vi "Pumps_Valves_Dependencies.vi"(8 "Set state:":bool, 10 "Device":T1=enum."V7") -> (0 "State":bool)   [LabVIEW 2011]
uses:
  Valve_Pump.ctl
  Pumps_Valves_Dependencies_Global.vi
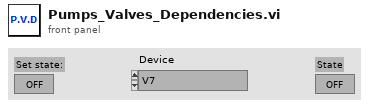
[diagram p1: front panel]
types:
  T1 = typedef "Valve_Pump.ctl" = enum16{"Main Rack Power", "Pump Power", "Valve Power", "V4", "V5", "V6", "V7", "V8", "V9", "V10", "V11", "V12", "V13", "V14", "V15", "V18", "V19", "V20", "V21", "V22", "V23", "V24", "V25", "V26", "V27", "V28", "V29", "V30", "V31", "V32", "V33", "V34", "Pump A", "Pump B", "Pump C", "Pump D"}
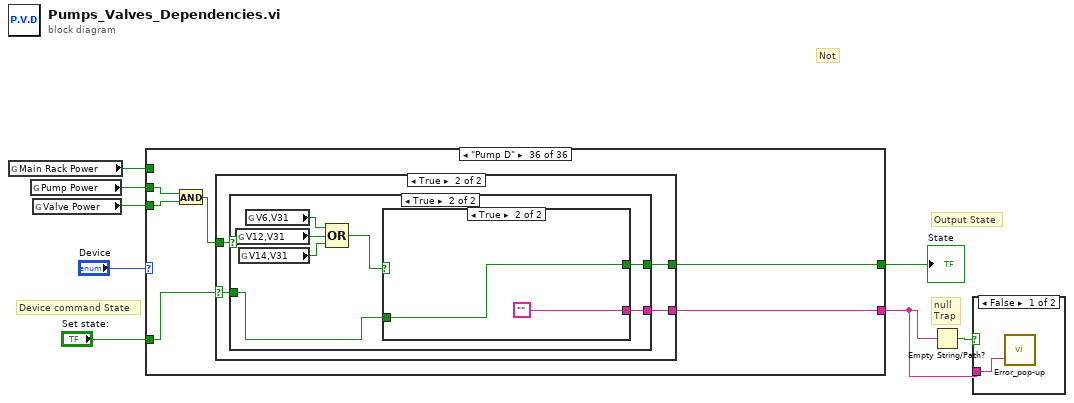
[diagram p0: block diagram]
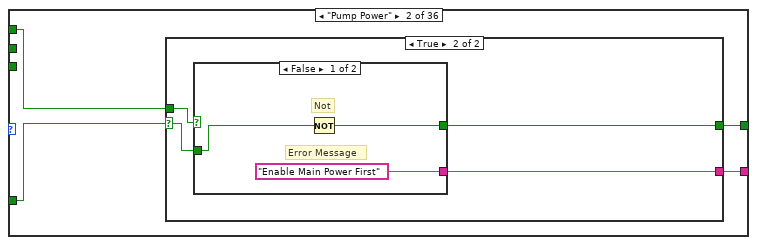
[diagram p4: hidden frame]
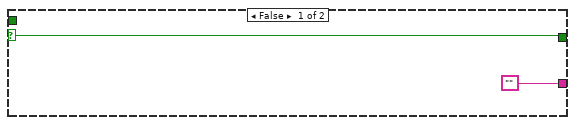
[diagram p5: hidden frame]
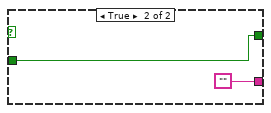
[diagram p6: hidden frame]
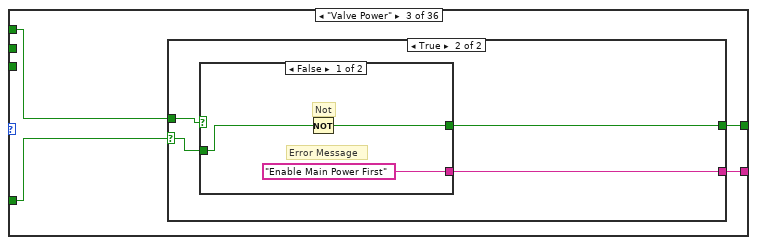
[diagram p7: hidden frame]
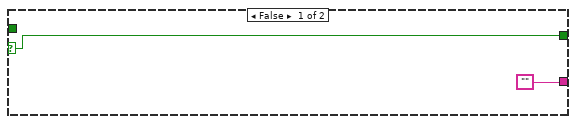
[diagram p8: hidden frame]
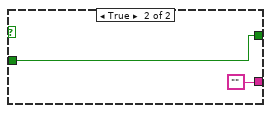
[diagram p9: hidden frame]
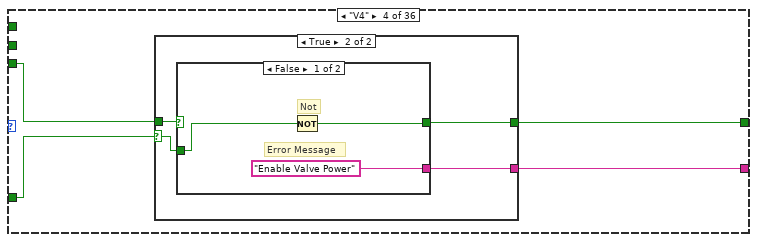
[diagram p10: hidden frame]
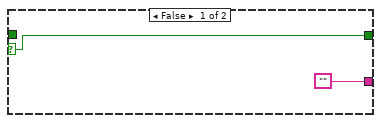
[diagram p11: hidden frame]
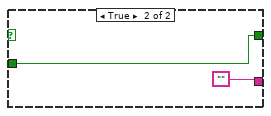
[diagram p12: hidden frame]
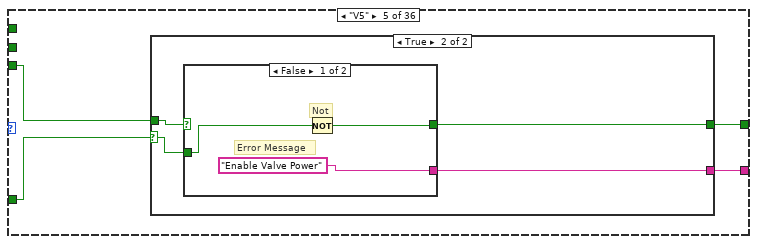
[diagram p13: hidden frame]
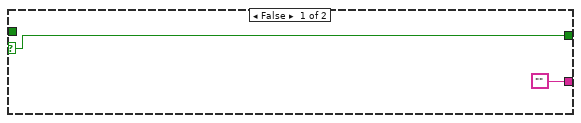
[diagram p14: hidden frame]
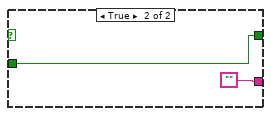
[diagram p15: hidden frame]
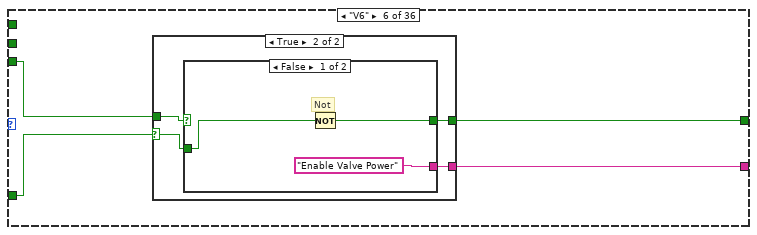
[diagram p16: hidden frame]
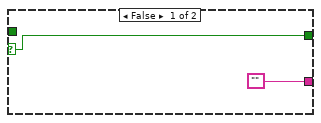
[diagram p17: hidden frame]
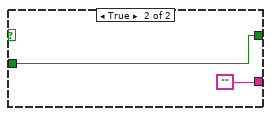
[diagram p18: hidden frame]
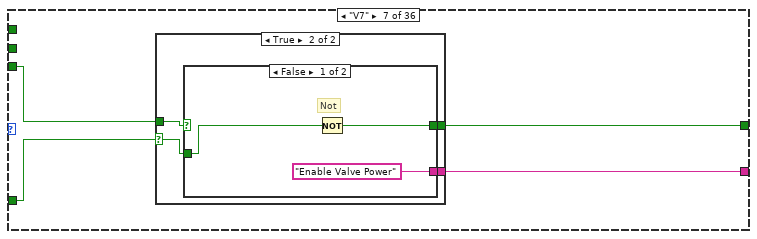
[diagram p19: hidden frame]
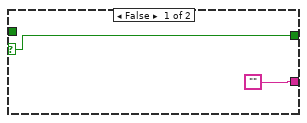
[diagram p20: hidden frame]
diagram:
  # "null\nTrap"
  # "Not"
  # "Device command State"
  # "Output State"
  n1 = global read "Pumps_Valves_Dependencies_Global.vi" "Main Rack Power"() -> (w3:bool)
  n2 = global read "Pumps_Valves_Dependencies_Global.vi" "Pump Power"() -> (w2:bool)
  n3 = global read "Pumps_Valves_Dependencies_Global.vi" "Valve Power"() -> (w1:bool)
  n4 = case shown="\"Pump D\"" "Device" {
    tunnel: "Set state:" -> [w9 w10 w25 w40 w55 w70 w85 w100 w115 w130 w145 w160 w175 w190 w205 w220 w235 w250 w265 w280 w295 w310 w325 w340 w355 w370 w385 w400 w415 w430 w445 w460 w475 w503 w530 w556]
    tunnel: [w9 w13 w27 w43 w58 w73 w88 w103 w118 w133 w148 w163 w178 w193 w208 w223 w238 w253 w268 w283 w298 w313 w328 w343 w358 w373 w388 w403 w418 w433 w448 w463 w477 w508 w533 w558] -> w6
    tunnel: [_ w12 w28 w42 w57 w72 w87 w102 w117 w132 w147 w162 w177 w192 w207 w222 w237 w252 w267 w282 w297 w312 w327 w342 w357 w372 w387 w402 w417 w432 w447 w462 w480 w507 w532 w559] -> w4
    tunnel: w3 -> [_ w11 w26 _ _ _ _ _ _ _ _ _ _ _ _ _ _ _ _ _ _ _ _ _ _ _ _ _ _ _ _ _ _ _ _ _]
    tunnel: w2 -> [_ _ _ _ _ _ _ _ _ _ _ _ _ _ _ _ _ _ _ _ _ _ _ _ _ _ _ _ _ _ _ _ w478 w505 w535 w561]
    tunnel: w1 -> [_ _ _ w41 w56 w71 w86 w101 w116 w131 w146 w161 w176 w191 w206 w221 w236 w251 w266 w281 w296 w311 w326 w341 w356 w371 w386 w401 w416 w431 w446 w461 w479 w506 w534 w560]
    frame "Main Rack Power" {
    }
    frame "Pump Power" {
      n5 = case shown="True" w10 {
        selector: w10 -> [w15 w16]
        tunnel: [w15 w19] -> w13
        tunnel: ["" w18] -> w12
        tunnel: w11 -> [_ w17]
        frame False {
        }
        frame True {
          n6 = case shown="False" w17 {
            tunnel: [w20 w24] -> w19
            tunnel: w16 -> [w21 w24]
            tunnel: ["Enable Main Power First" ""] -> w18
            frame False {
              # "Error Message"
              # "Not"
              n7 = Not(x=w21) -> (.not. x?=w20:bool)
            }
            frame True {
            }
          }
        }
      }
    }
    frame "Valve Power" {
      n8 = case shown="True" w25 {
        selector: w25 -> [w30 w31]
        tunnel: ["" w34] -> w28
        tunnel: [w30 w33] -> w27
        tunnel: w26 -> [_ w32]
        frame False {
        }
        frame True {
          n9 = case shown="False" w32 {
            tunnel: [w35 w39] -> w33
            tunnel: w31 -> [w36 w39]
            tunnel: ["Enable Main Power First" ""] -> w34
            frame False {
              # "Error Message"
              # "Not"
              n10 = Not(x=w36) -> (.not. x?=w35:bool)
            }
            frame True {
            }
          }
        }
      }
    }
    frame "V4" {
      n11 = case shown="True" w40 {
        selector: w40 -> [w45 w46]
        tunnel: [w45 w49] -> w43
        tunnel: ["" w48] -> w42
        tunnel: w41 -> [_ w47]
        frame False {
        }
        frame True {
          n12 = case shown="False" w47 {
            tunnel: [w50 w54] -> w49
            tunnel: w46 -> [w51 w54]
            tunnel: ["Enable Valve Power" ""] -> w48
            frame False {
              # "Not"
              # "Error Message"
              n13 = Not(x=w51) -> (.not. x?=w50:bool)
            }
            frame True {
            }
          }
        }
      }
    }
    frame "V5" {
      n14 = case shown="True" w55 {
        selector: w55 -> [w60 w61]
        tunnel: [w60 w64] -> w58
        tunnel: ["" w63] -> w57
        tunnel: w56 -> [_ w62]
        frame False {
        }
        frame True {
          n15 = case shown="False" w62 {
            tunnel: [w66 w69] -> w64
            tunnel: w61 -> [w65 w69]
            tunnel: ["Enable Valve Power" ""] -> w63
            frame False {
              # "Error Message"
              # "Not"
              n16 = Not(x=w65) -> (.not. x?=w66:bool)
            }
            frame True {
            }
          }
        }
      }
    }
    frame "V6" {
      n17 = case shown="True" w70 {
        selector: w70 -> [w75 w76]
        tunnel: [w75 w79] -> w73
        tunnel: ["" w78] -> w72
        tunnel: w71 -> [_ w77]
        frame False {
        }
        frame True {
          n18 = case shown="False" w77 {
            tunnel: [w81 w84] -> w79
            tunnel: w76 -> [w80 w84]
            tunnel: ["Enable Valve Power" ""] -> w78
            frame False {
              # "Not"
              n19 = Not(x=w80) -> (.not. x?=w81:bool)
            }
            frame True {
            }
          }
        }
      }
    }
    frame "V7" {
      n20 = case shown="True" w85 {
        selector: w85 -> [w90 w91]
        tunnel: [w90 w94] -> w88
        tunnel: ["" w93] -> w87
        tunnel: w86 -> [_ w92]
        frame False {
        }
        frame True {
          n21 = case shown="False" w92 {
            tunnel: [w96 w99] -> w94
            tunnel: w91 -> [w95 w99]
            tunnel: ["Enable Valve Power" ""] -> w93
            frame False {
              # "Not"
              n22 = Not(x=w95) -> (.not. x?=w96:bool)
            }
            frame True {
            }
          }
        }
      }
    }
    frame "V8" {
      n23 = case shown="True" w100 {
        selector: w100 -> [w104 w106]
        tunnel: [w104 w109] -> w103
        tunnel: ["" w108] -> w102
        tunnel: w101 -> [_ w107]
        frame False {
        }
        frame True {
          n24 = case shown="False" w107 {
            tunnel: [w110 w114] -> w109
            tunnel: w106 -> [w111 w114]
            tunnel: ["Enable Valve Power" ""] -> w108
            frame False {
              # "Not"
              n25 = Not(x=w111) -> (.not. x?=w110:bool)
            }
            frame True {
            }
          }
        }
      }
    }
    frame "V9" {
      n26 = case shown="True" w115 {
        selector: w115 -> [w120 w121]
        tunnel: [w120 w124] -> w118
        tunnel: ["" w123] -> w117
        tunnel: w116 -> [_ w122]
        frame False {
        }
        frame True {
          n27 = case shown="False" w122 {
            tunnel: [w126 w129] -> w124
            tunnel: w121 -> [w125 w129]
            tunnel: ["Enable Valve Power" ""] -> w123
            frame False {
              # "Not"
              n28 = Not(x=w125) -> (.not. x?=w126:bool)
            }
            frame True {
            }
          }
        }
      }
    }
    frame "V10" {
      n29 = case shown="True" w130 {
        selector: w130 -> [w135 w136]
        tunnel: [w135 w139] -> w133
        tunnel: ["" w138] -> w132
        tunnel: w131 -> [_ w137]
        frame False {
        }
        frame True {
          n30 = case shown="False" w137 {
            tunnel: [w140 w144] -> w139
            tunnel: w136 -> [w141 w144]
            tunnel: ["Enable Valve Power" ""] -> w138
            frame False {
              # "Not"
              n31 = Not(x=w141) -> (.not. x?=w140:bool)
            }
            frame True {
            }
          }
        }
      }
    }
    frame "V11" {
      n32 = case shown="True" w145 {
        selector: w145 -> [w150 w151]
        tunnel: [w150 w154] -> w148
        tunnel: ["" w153] -> w147
        tunnel: w146 -> [_ w152]
        frame False {
        }
        frame True {
          n33 = case shown="False" w152 {
            tunnel: [w155 w159] -> w154
            tunnel: w151 -> [w156 w159]
            tunnel: ["Enable Valve Power" ""] -> w153
            frame False {
              # "Not"
              n34 = Not(x=w156) -> (.not. x?=w155:bool)
            }
            frame True {
            }
          }
        }
      }
    }
    frame "V12" {
      n35 = case shown="True" w160 {
        selector: w160 -> [w164 w166]
        tunnel: [w164 w169] -> w163
        tunnel: ["" w168] -> w162
        tunnel: w161 -> [_ w167]
        frame False {
        }
        frame True {
          n36 = case shown="False" w167 {
            tunnel: [w171 w174] -> w169
            tunnel: w166 -> [w170 w174]
            tunnel: ["Enable Valve Power" ""] -> w168
            frame False {
              # "Not"
              n37 = Not(x=w170) -> (.not. x?=w171:bool)
            }
            frame True {
            }
          }
        }
      }
    }
    frame "V13" {
      n38 = case shown="True" w175 {
        selector: w175 -> [w180 w181]
        tunnel: [w180 w184] -> w178
        tunnel: ["" w183] -> w177
        tunnel: w176 -> [_ w182]
        frame False {
        }
        frame True {
          n39 = case shown="False" w182 {
            tunnel: [w186 w189] -> w184
            tunnel: w181 -> [w185 w189]
            tunnel: ["Enable Valve Power" ""] -> w183
            frame False {
              # "Not"
              n40 = Not(x=w185) -> (.not. x?=w186:bool)
            }
            frame True {
            }
          }
        }
      }
    }
    frame "V14" {
      n41 = case shown="True" w190 {
        selector: w190 -> [w194 w196]
        tunnel: [w194 w199] -> w193
        tunnel: ["" w198] -> w192
        tunnel: w191 -> [_ w197]
        frame False {
        }
        frame True {
          n42 = case shown="False" w197 {
            tunnel: [w200 w204] -> w199
            tunnel: w196 -> [w201 w204]
            tunnel: ["Enable Valve Power" ""] -> w198
            frame False {
              # "Not"
              n43 = Not(x=w201) -> (.not. x?=w200:bool)
            }
            frame True {
            }
          }
        }
      }
    }
    frame "V15" {
      n44 = case shown="True" w205 {
        selector: w205 -> [w210 w211]
        tunnel: [w210 w214] -> w208
        tunnel: ["" w213] -> w207
        tunnel: w206 -> [_ w212]
        frame False {
        }
        frame True {
          n45 = case shown="False" w212 {
            tunnel: [w215 w219] -> w214
            tunnel: w211 -> [w216 w219]
            tunnel: ["Enable Valve Power" ""] -> w213
            frame False {
              # "Not"
              n46 = Not(x=w216) -> (.not. x?=w215:bool)
            }
            frame True {
            }
          }
        }
      }
    }
    frame "V18" {
      n47 = case shown="True" w220 {
        selector: w220 -> [w225 w226]
        tunnel: [w225 w229] -> w223
        tunnel: ["" w228] -> w222
        tunnel: w221 -> [_ w227]
        frame False {
        }
        frame True {
          n48 = case shown="False" w227 {
            tunnel: [w231 w234] -> w229
            tunnel: w226 -> [w230 w234]
            tunnel: ["Enable Valve Power" ""] -> w228
            frame False {
              # "Not"
              n49 = Not(x=w230) -> (.not. x?=w231:bool)
            }
            frame True {
            }
          }
        }
      }
    }
    frame "V19" {
      n50 = case shown="True" w235 {
        selector: w235 -> [w240 w241]
        tunnel: [w240 w244] -> w238
        tunnel: ["" w243] -> w237
        tunnel: w236 -> [_ w242]
        frame False {
        }
        frame True {
          n51 = case shown="False" w242 {
            tunnel: [w246 w249] -> w244
            tunnel: w241 -> [w245 w249]
            tunnel: ["Enable Valve Power" ""] -> w243
            frame False {
              # "Not"
              n52 = Not(x=w245) -> (.not. x?=w246:bool)
            }
            frame True {
            }
          }
        }
      }
    }
    frame "V20" {
      n53 = case shown="True" w250 {
        selector: w250 -> [w255 w256]
        tunnel: [w255 w259] -> w253
        tunnel: ["" w258] -> w252
        tunnel: w251 -> [_ w257]
        frame False {
        }
        frame True {
          n54 = case shown="False" w257 {
            tunnel: [w261 w264] -> w259
            tunnel: w256 -> [w260 w264]
            tunnel: ["Enable Valve Power" ""] -> w258
            frame False {
              # "Not"
              n55 = Not(x=w260) -> (.not. x?=w261:bool)
            }
            frame True {
            }
          }
        }
      }
    }
    frame "V21" {
      n56 = case shown="True" w265 {
        selector: w265 -> [w270 w271]
        tunnel: [w270 w274] -> w268
        tunnel: ["" w273] -> w267
        tunnel: w266 -> [_ w272]
        frame False {
        }
        frame True {
          n57 = case shown="False" w272 {
            tunnel: [w276 w279] -> w274
            tunnel: w271 -> [w275 w279]
            tunnel: ["Enable Valve Power" ""] -> w273
            frame False {
              # "Not"
              n58 = Not(x=w275) -> (.not. x?=w276:bool)
            }
            frame True {
            }
          }
        }
      }
    }
    frame "V22" {
      n59 = case shown="True" w280 {
        selector: w280 -> [w285 w286]
        tunnel: [w285 w289] -> w283
        tunnel: ["" w288] -> w282
        tunnel: w281 -> [_ w287]
        frame False {
        }
        frame True {
          n60 = case shown="False" w287 {
            tunnel: [w291 w294] -> w289
            tunnel: w286 -> [w290 w294]
            tunnel: ["Enable Valve Power" ""] -> w288
            frame False {
              # "Not"
              n61 = Not(x=w290) -> (.not. x?=w291:bool)
            }
            frame True {
            }
          }
        }
      }
    }
    frame "V23" {
      n62 = case shown="True" w295 {
        selector: w295 -> [w300 w301]
        tunnel: [w300 w304] -> w298
        tunnel: ["" w303] -> w297
        tunnel: w296 -> [_ w302]
        frame False {
        }
        frame True {
          n63 = case shown="False" w302 {
            tunnel: [w306 w309] -> w304
            tunnel: w301 -> [w305 w309]
            tunnel: ["Enable Valve Power" ""] -> w303
            frame False {
              # "Not"
              n64 = Not(x=w305) -> (.not. x?=w306:bool)
            }
            frame True {
            }
          }
        }
      }
    }
    frame "V24" {
      n65 = case shown="True" w310 {
        selector: w310 -> [w315 w316]
        tunnel: [w315 w319] -> w313
        tunnel: ["" w318] -> w312
        tunnel: w311 -> [_ w317]
        frame False {
        }
        frame True {
          n66 = case shown="False" w317 {
            tunnel: [w321 w324] -> w319
            tunnel: w316 -> [w320 w324]
            tunnel: ["Enable Valve Power" ""] -> w318
            frame False {
              # "Not"
              n67 = Not(x=w320) -> (.not. x?=w321:bool)
            }
            frame True {
            }
          }
        }
      }
    }
    frame "V25" {
      n68 = case shown="True" w325 {
        selector: w325 -> [w330 w331]
        tunnel: [w330 w334] -> w328
        tunnel: ["" w333] -> w327
        tunnel: w326 -> [_ w332]
        frame False {
        }
        frame True {
          n69 = case shown="False" w332 {
            tunnel: [w336 w339] -> w334
            tunnel: w331 -> [w335 w339]
            tunnel: ["Enable Valve Power" ""] -> w333
            frame False {
              # "Not"
              n70 = Not(x=w335) -> (.not. x?=w336:bool)
            }
            frame True {
            }
          }
        }
      }
    }
    frame "V26" {
      n71 = case shown="True" w340 {
        selector: w340 -> [w345 w346]
        tunnel: [w345 w349] -> w343
        tunnel: ["" w348] -> w342
        tunnel: w341 -> [_ w347]
        frame False {
        }
        frame True {
          n72 = case shown="False" w347 {
            tunnel: [w351 w354] -> w349
            tunnel: w346 -> [w350 w354]
            tunnel: ["Enable Valve Power" ""] -> w348
            frame False {
              # "Not"
              n73 = Not(x=w350) -> (.not. x?=w351:bool)
            }
            frame True {
            }
          }
        }
      }
    }
    frame "V27" {
      n74 = case shown="True" w355 {
        selector: w355 -> [w360 w361]
        tunnel: [w360 w364] -> w358
        tunnel: ["" w363] -> w357
        tunnel: w356 -> [_ w362]
        frame False {
        }
        frame True {
          n75 = case shown="False" w362 {
            tunnel: [w366 w369] -> w364
            tunnel: w361 -> [w365 w369]
            tunnel: ["Enable Valve Power" ""] -> w363
            frame False {
              # "Not"
              n76 = Not(x=w365) -> (.not. x?=w366:bool)
            }
            frame True {
            }
          }
        }
      }
    }
    frame "V28" {
      n77 = case shown="True" w370 {
        selector: w370 -> [w375 w376]
        tunnel: [w375 w379] -> w373
        tunnel: ["" w378] -> w372
        tunnel: w371 -> [_ w377]
        frame False {
        }
        frame True {
          n78 = case shown="False" w377 {
            tunnel: [w381 w384] -> w379
            tunnel: w376 -> [w380 w384]
            tunnel: ["Enable Valve Power" ""] -> w378
            frame False {
              # "Not"
              n79 = Not(x=w380) -> (.not. x?=w381:bool)
            }
            frame True {
            }
          }
        }
      }
    }
    frame "V29" {
      n80 = case shown="True" w385 {
        selector: w385 -> [w390 w391]
        tunnel: [w390 w394] -> w388
        tunnel: ["" w393] -> w387
        tunnel: w386 -> [_ w392]
        frame False {
        }
        frame True {
          n81 = case shown="False" w392 {
            tunnel: [w396 w399] -> w394
            tunnel: w391 -> [w395 w399]
            tunnel: ["Enable Valve Power" ""] -> w393
            frame False {
              # "Not"
              n82 = Not(x=w395) -> (.not. x?=w396:bool)
            }
            frame True {
            }
          }
        }
      }
    }
    frame "V30" {
      n83 = case shown="True" w400 {
        selector: w400 -> [w405 w406]
        tunnel: [w405 w409] -> w403
        tunnel: ["" w408] -> w402
        tunnel: w401 -> [_ w407]
        frame False {
        }
        frame True {
          n84 = case shown="False" w407 {
            tunnel: [w411 w414] -> w409
            tunnel: w406 -> [w410 w414]
            tunnel: ["Enable Valve Power" ""] -> w408
            frame False {
              # "Not"
              n85 = Not(x=w410) -> (.not. x?=w411:bool)
            }
            frame True {
            }
          }
        }
      }
    }
    frame "V31" {
      n86 = case shown="True" w415 {
        selector: w415 -> [w420 w421]
        tunnel: [w420 w424] -> w418
        tunnel: ["" w423] -> w417
        tunnel: w416 -> [_ w422]
        frame False {
        }
        frame True {
          n87 = case shown="False" w422 {
            tunnel: [w426 w429] -> w424
            tunnel: w421 -> [w425 w429]
            tunnel: ["Enable Valve Power" ""] -> w423
            frame False {
              # "Not"
              n88 = Not(x=w425) -> (.not. x?=w426:bool)
            }
            frame True {
            }
          }
        }
      }
    }
    frame "V32" {
      n89 = case shown="True" w430 {
        selector: w430 -> [w435 w436]
        tunnel: [w435 w439] -> w433
        tunnel: ["" w438] -> w432
        tunnel: w431 -> [_ w437]
        frame False {
        }
        frame True {
          n90 = case shown="False" w437 {
            tunnel: [w441 w444] -> w439
            tunnel: w436 -> [w440 w444]
            tunnel: ["Enable Valve Power" ""] -> w438
            frame False {
              # "Not"
              n91 = Not(x=w440) -> (.not. x?=w441:bool)
            }
            frame True {
            }
          }
        }
      }
    }
    frame "V33" {
      n92 = case shown="True" w445 {
        selector: w445 -> [w450 w451]
        tunnel: [w450 w454] -> w448
        tunnel: ["" w453] -> w447
        tunnel: w446 -> [_ w452]
        frame False {
        }
        frame True {
          n93 = case shown="False" w452 {
            tunnel: [w456 w459] -> w454
            tunnel: w451 -> [w455 w459]
            tunnel: ["Enable Valve Power" ""] -> w453
            frame False {
              # "Not"
              n94 = Not(x=w455) -> (.not. x?=w456:bool)
            }
            frame True {
            }
          }
        }
      }
    }
    frame "V34" {
      n95 = case shown="True" w460 {
        selector: w460 -> [w465 w466]
        tunnel: [w465 w469] -> w463
        tunnel: ["" w468] -> w462
        tunnel: w461 -> [_ w467]
        frame False {
        }
        frame True {
          n96 = case shown="False" w467 {
            tunnel: [w471 w474] -> w469
            tunnel: w466 -> [w470 w474]
            tunnel: ["Enable Valve Power" ""] -> w468
            frame False {
              # "Not"
              n97 = Not(x=w470) -> (.not. x?=w471:bool)
            }
            frame True {
            }
          }
        }
      }
    }
    frame "Pump A" {
      n98 = And(x=w478, y=w479) -> (x .and. y?=w476:bool)
      n99 = case shown="True" w475 {
        selector: w475 -> [w482 w483]
        tunnel: ["" w485] -> w480
        tunnel: [w482 w486] -> w477
        tunnel: w476 -> [_ w484]
        frame False {
        }
        frame True {
          n100 = case shown="True" w484 {
            tunnel: [w487 w496] -> w486
            tunnel: ["Enable Pump Power\n and  Valve Power" w495] -> w485
            tunnel: w483 -> [w488 w491]
            frame False {
              n101 = Not(x=w488) -> (.not. x?=w487:bool)
            }
            frame True {
              n102 = global read "Pumps_Valves_Dependencies_Global.vi" "V29,V28"() -> (w494:bool)
              n103 = global read "Pumps_Valves_Dependencies_Global.vi" "V29,V27"() -> (w493:bool)
              n104 = global read "Pumps_Valves_Dependencies_Global.vi" "V29,V23"() -> (w492:bool)
              n105 = global read "Pumps_Valves_Dependencies_Global.vi" "V30,V28"() -> (w490:bool)
              n106 = Compound Arithmetic op=OR(w494, w493, w492, w490) -> (w497:bool)
              n107 = case shown="False" w497 {
                tunnel: ["Enable V29 along with \nV28 or V27 or V23.\n Alternatively V30 and\nV29" ""] -> w495
                tunnel: w491 -> [w499 w502]
                tunnel: [w498 w502] -> w496
                frame False {
                  # "Not"
                  n108 = Not(x=w499) -> (.not. x?=w498:bool)
                }
                frame True {
                }
              }
            }
          }
        }
      }
    }
    frame "Pump B" {
      n109 = And(x=w505, y=w506) -> (x .and. y?=w504:bool)
      n110 = case shown="True" w503 {
        selector: w503 -> [w510 w511]
        tunnel: ["" w513] -> w507
        tunnel: [w510 w514] -> w508
        tunnel: w504 -> [_ w512]
        frame False {
        }
        frame True {
          n111 = case shown="True" w512 {
            tunnel: [w515 w523] -> w514
            tunnel: ["Enable Pump Power\n and  Valve Power" w522] -> w513
            tunnel: w511 -> [w516 w519]
            frame False {
              # "Not"
              n112 = Not(x=w516) -> (.not. x?=w515:bool)
            }
            frame True {
              n113 = global read "Pumps_Valves_Dependencies_Global.vi" "V4,V33,V19"() -> (w520:bool)
              n114 = global read "Pumps_Valves_Dependencies_Global.vi" "V5,V33,V19"() -> (w521:bool)
              n115 = global read "Pumps_Valves_Dependencies_Global.vi" "V9,V15,V33"() -> (w518:bool)
              n116 = Compound Arithmetic op=OR(w520, w521, w518) -> (w524:bool)
              n117 = case shown="False" w524 {
                tunnel: ["Enable V33 and V19\nalong with V4 or V5" ""] -> w522
                tunnel: w519 -> [w526 w529]
                tunnel: [w525 w529] -> w523
                frame False {
                  # "Not"
                  n118 = Not(x=w526) -> (.not. x?=w525:bool)
                }
                frame True {
                }
              }
            }
          }
        }
      }
    }
    frame "Pump C" {
      n119 = And(x=w535, y=w534) -> (x .and. y?=w531:bool)
      n120 = case shown="True" w530 {
        selector: w530 -> [w537 w538]
        tunnel: ["" w541] -> w532
        tunnel: [w537 w540] -> w533
        tunnel: w531 -> [_ w539]
        frame False {
        }
        frame True {
          n121 = case shown="True" w539 {
            tunnel: ["Enable Pump Power\n and  Valve Power" w549] -> w541
            tunnel: [w542 w548] -> w540
            tunnel: w538 -> [w543 w545]
            frame False {
              # "Not"
              n122 = Not(x=w543) -> (.not. x?=w542:bool)
            }
            frame True {
              n123 = global read "Pumps_Valves_Dependencies_Global.vi" "V7,V19/V18"() -> (w546:bool)
              n124 = global read "Pumps_Valves_Dependencies_Global.vi" "V9,V13,V19"() -> (w547:bool)
              n125 = Compound Arithmetic op=OR(w546, w547) -> (w550:bool)
              n126 = case shown="False" w550 {
                tunnel: ["During filling (V19 open), to get fresh water from Tank C, enable V19 or V18 along with V7. Alternatively to get fresh water from Tank D, enable V9, V13 and V19." ""] -> w549
                tunnel: w545 -> [w552 w555]
                tunnel: [w551 w555] -> w548
                frame False {
                  # "Not"
                  n127 = Not(x=w552) -> (.not. x?=w551:bool)
                }
                frame True {
                }
              }
            }
          }
        }
      }
    }
    frame "Pump D" {
      n128 = And(x=w561, y=w560) -> (x .and. y?=w557:bool)
      n129 = case shown="True" w556 {
        selector: w556 -> [w563 w564]
        tunnel: ["" w567] -> w559
        tunnel: [w563 w566] -> w558
        tunnel: w557 -> [_ w565]
        frame False {
        }
        frame True {
          n130 = case shown="True" w565 {
            tunnel: ["Enable Pump Power\n and  Valve Power" w576] -> w567
            tunnel: [w568 w575] -> w566
            tunnel: w564 -> [w569 w571]
            frame False {
              n131 = Not(x=w569) -> (.not. x?=w568:bool)
            }
            frame True {
              n132 = global read "Pumps_Valves_Dependencies_Global.vi" "V12,V31"() -> (w573:bool)
              n133 = global read "Pumps_Valves_Dependencies_Global.vi" "V14,V31"() -> (w572:bool)
              n134 = global read "Pumps_Valves_Dependencies_Global.vi" "V6,V31"() -> (w574:bool)
              n135 = Compound Arithmetic op=OR(w574, w573, w572) -> (w577:bool)
              n136 = case shown="True" w577 {
                tunnel: ["Enable V31 along with V6 or V12 or V14" ""] -> w576
                tunnel: w571 -> [w579 w582]
                tunnel: [w578 w582] -> w575
                frame False {
                  n137 = Not(x=w579) -> (.not. x?=w578:bool)
                }
                frame True {
                }
              }
            }
          }
        }
      }
    }
  }
  "State" <- w6
  n138 = Empty String/Path?(string/path=w4) -> (empty?=w5:bool)
  n139 = case shown="False" w5 {
    tunnel: w4 -> [w583 _]
    frame False {
      n140 = call "Error_pop-up.vi"("New msg"=w583) -> ()  [unwired: 2 in]
    }
    frame True {
    }
  }
